vi "Piezo Message Loop.vi"(8 "error in (no error)":errorcluster, 10 "Data Notifiers":T2, 11 "Message Queues":T3) -> (0 "error out":errorcluster)   [LabVIEW 2013, in "Piezo.lvlib"]
uses:
  Piezo.lvlib
  support/Message Queue/All Message Queues.ctl
  support/Message Queue/Message Cluster.ctl
  support/Data Notifiers/All Data Notifiers.ctl
  Acquisition/APD Notifier Cluster.ctl
  Piezo display.ctl
  XY/XY Display.ctl
  Capacitive/Capacitive Signal Cluster.ctl
  Feedback/Error Signal.ctl
  piezo new/Hardware Configuration Piezo NEW.ctl
  Untitled Project 3 Andrea/piezo new/Hardware Configuration Piezo out.ctl
  Piezo State.ctl
  support/Message Queue/Enqueue Message (Single).vi
  <vilib>/Utility/error.llb/Error Cluster From Error Code.vi
  <vilib>/ErrorRing/Error Ring.xnode
  support/Message Queue/Message Queue.lvlib
  Acquisition/Acquisition.lvlib
  XY/XY.lvlib
  support/Data Notifiers/Data Notifiers.lvlib
  Capacitive/Capacitive.lvlib
  Feedback/Feedback.lvlib
panel:
  out "Numeric":i32
  in  "Cluster":T1
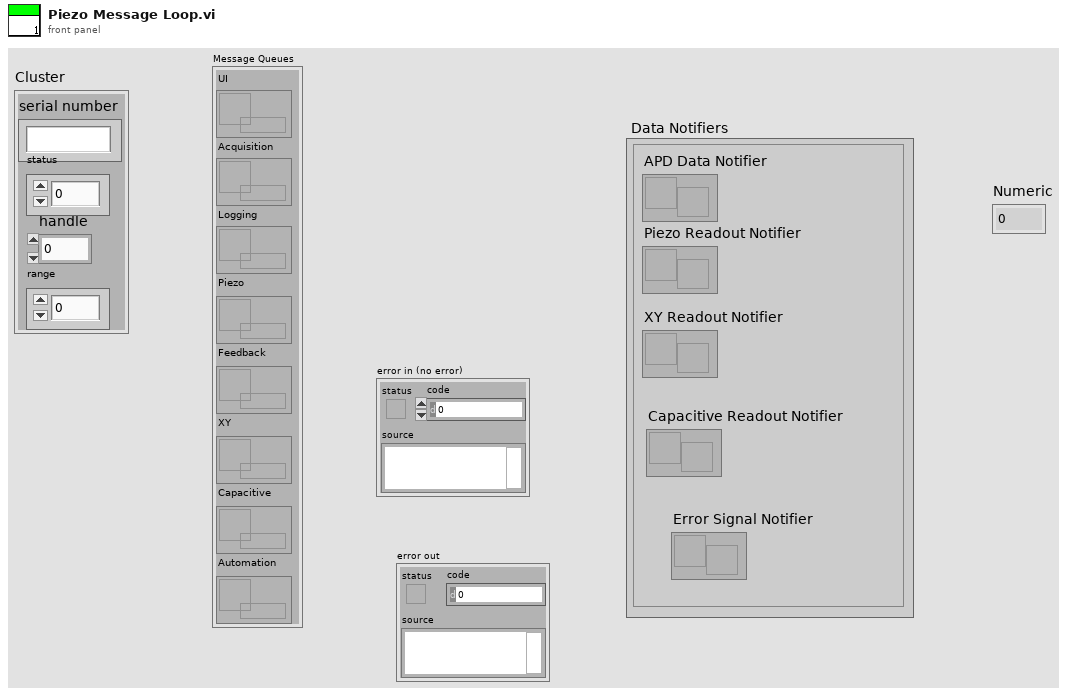
[diagram p1: front panel]
types:
  T1 = typedef "Hardware Configuration Piezo NEW.ctl" = cluster{"serial number":string, "handle":i32, "status":i32, "range":i32}
  T2 = typedef "Data Notifiers.lvlib/All Data Notifiers.ctl" = cluster{"APD Data Notifier":refnum<notifier>, "Piezo Readout Notifier":refnum<notifier>, "XY Readout Notifier":refnum<notifier>, "Capacitive Readout Notifier":refnum<notifier>, "Error Signal Notifier":refnum<notifier>}
  T3 = typedef "Message Queue.lvlib/All Message Queues.ctl" = cluster{"UI":refnum<queue>, "Acquisition":refnum<queue>, "Logging":refnum<queue>, "Piezo":refnum<queue>, "Feedback":refnum<queue>, "XY":refnum<queue>, "Capacitive":refnum<queue>, "Automation":refnum<queue>}
  T4 = typedef "Hardware Configuration Piezo out.ctl" = cluster{"physical channels":tag, "MAX   VOLTAGE":dbl, "MIN   VOLTAGE":dbl}
  T5 = typedef "Piezo.lvlib/Piezo State.ctl" = enum16{"Idle", "Acquiring"}
  T6 = typedef "Acquisition.lvlib/APD Notifier Cluster.ctl" = cluster{"data":dbl[][], "t0":i32}
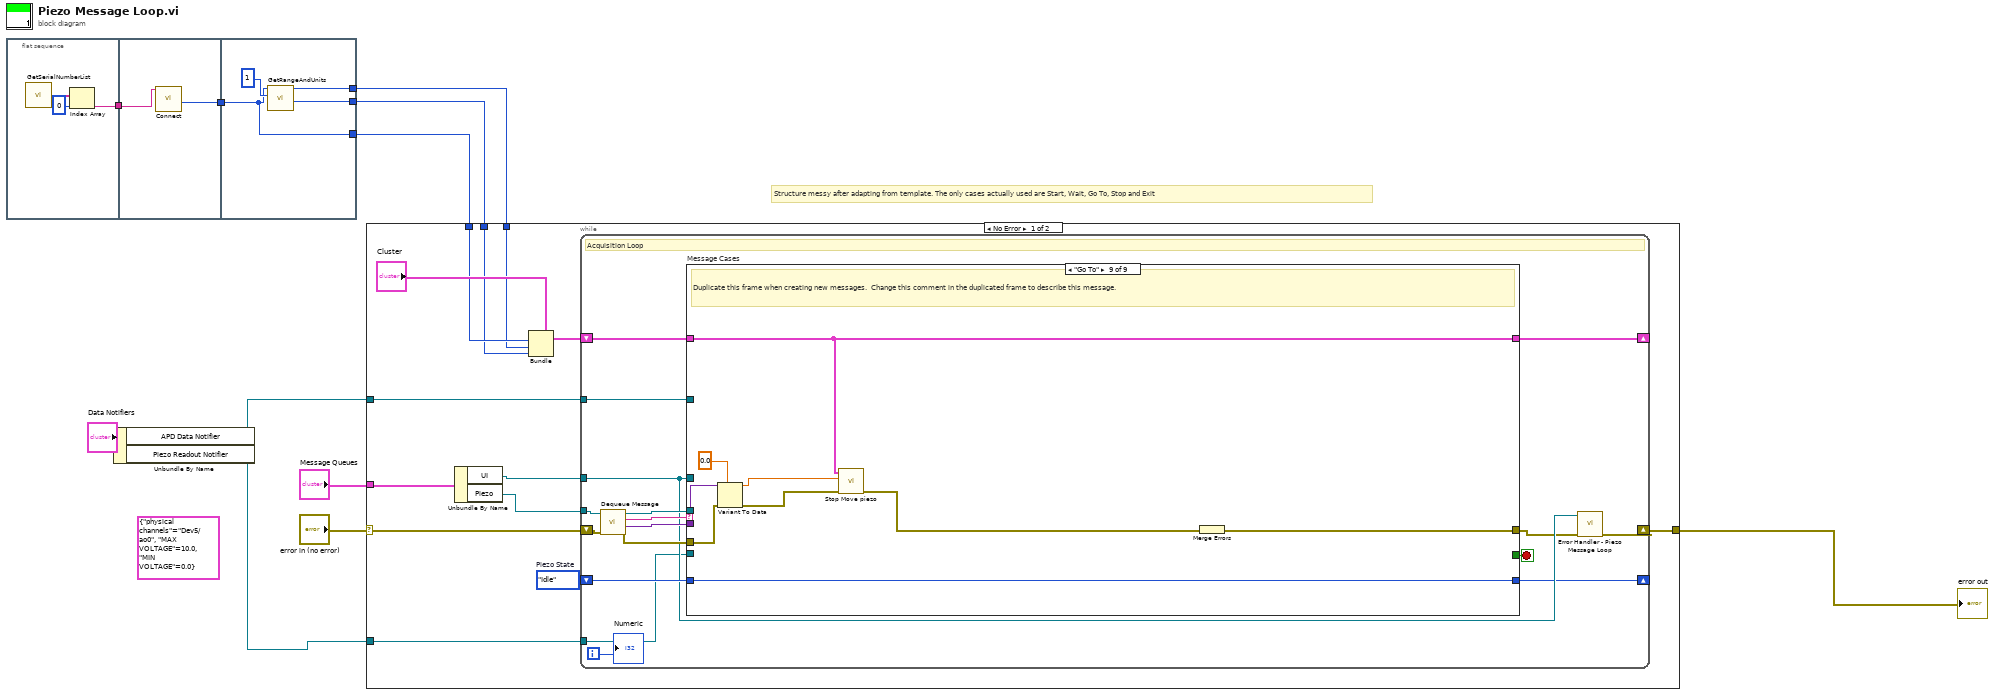
[diagram p0: block diagram]
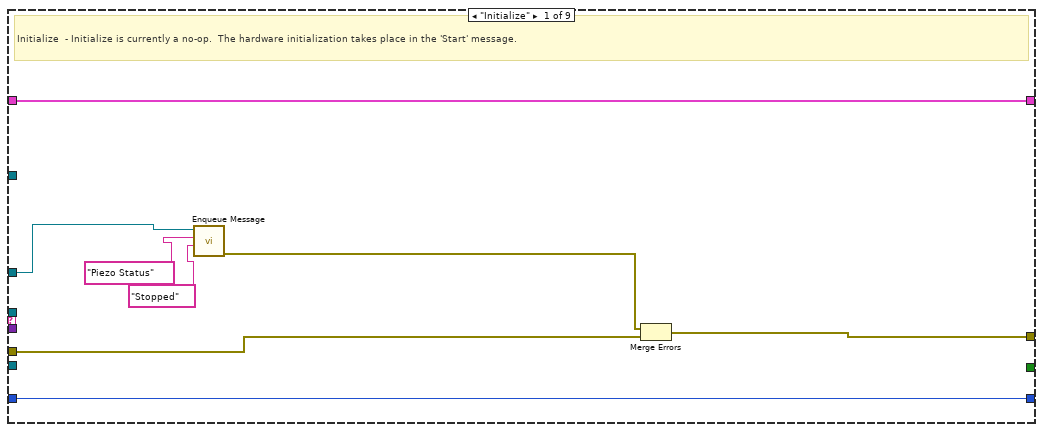
[diagram p2: hidden frame]
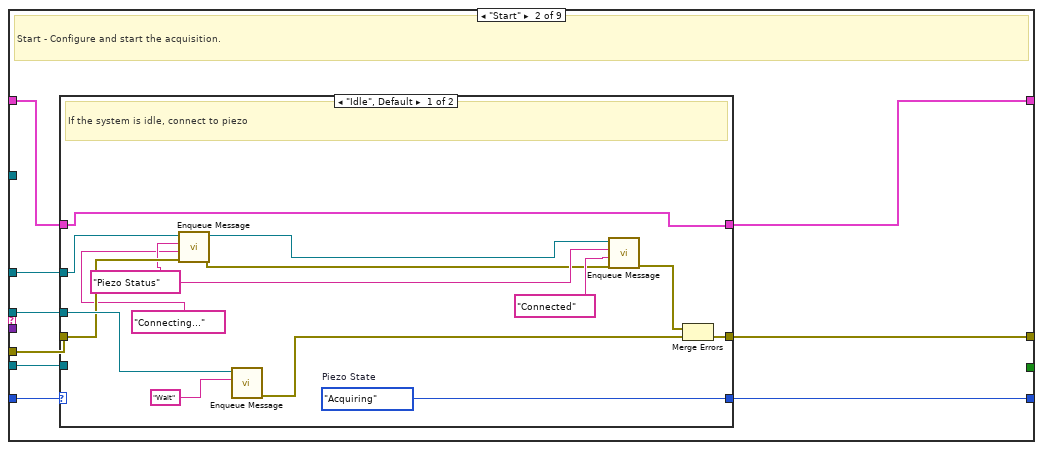
[diagram p3: hidden frame]
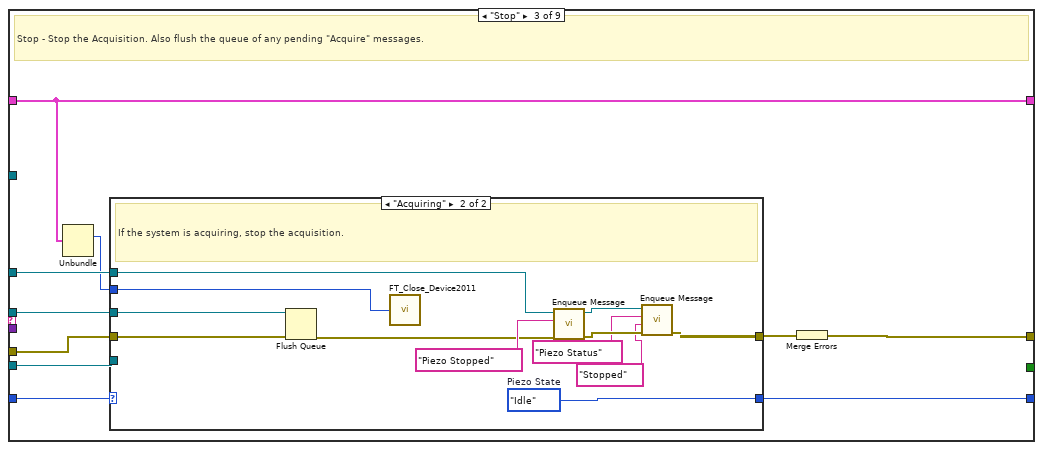
[diagram p5: hidden frame]
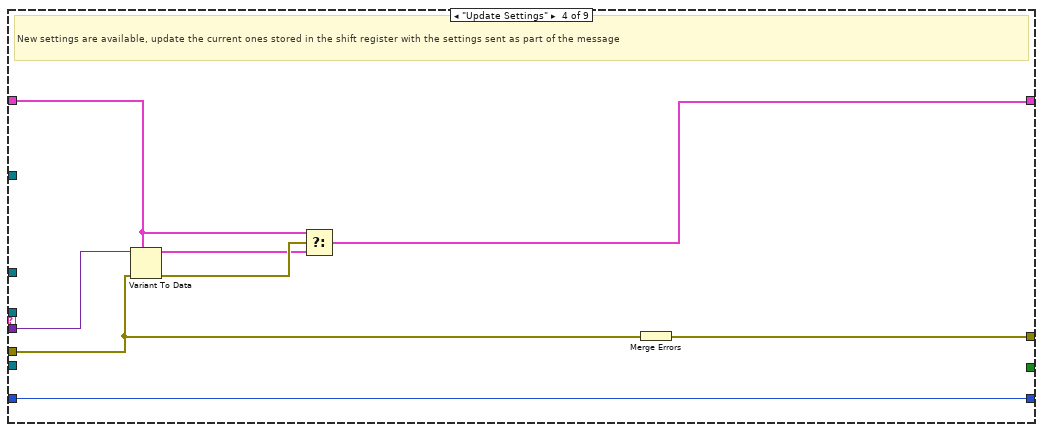
[diagram p7: hidden frame]
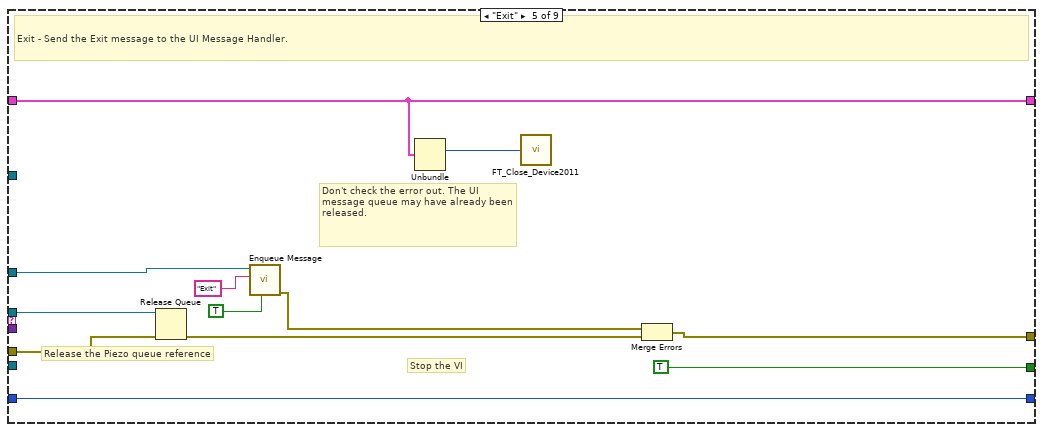
[diagram p8: hidden frame]
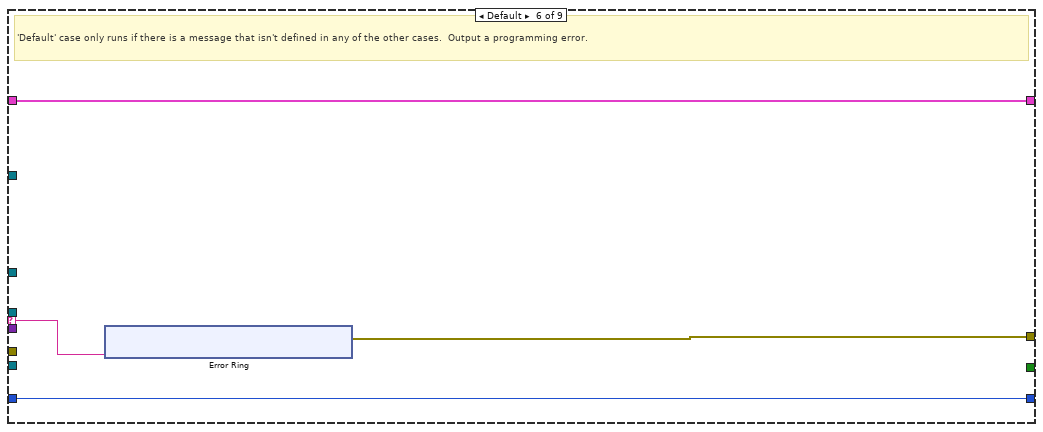
[diagram p9: hidden frame]
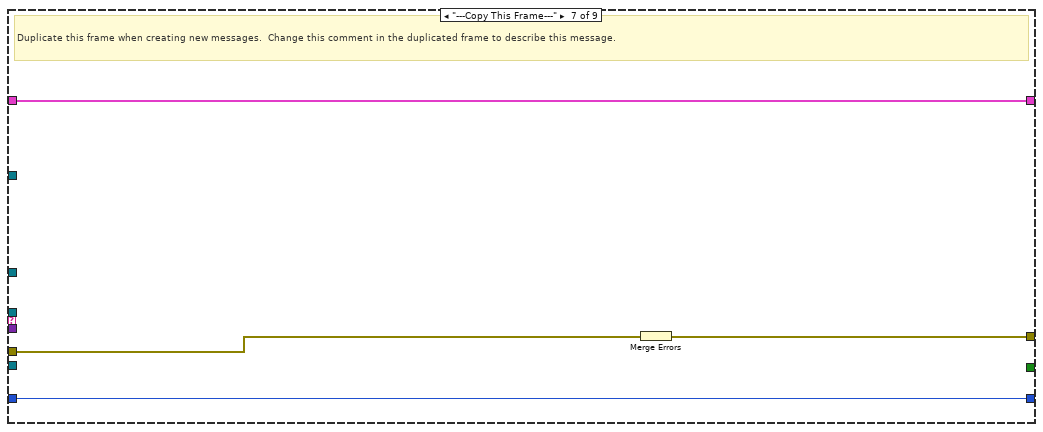
[diagram p10: hidden frame]
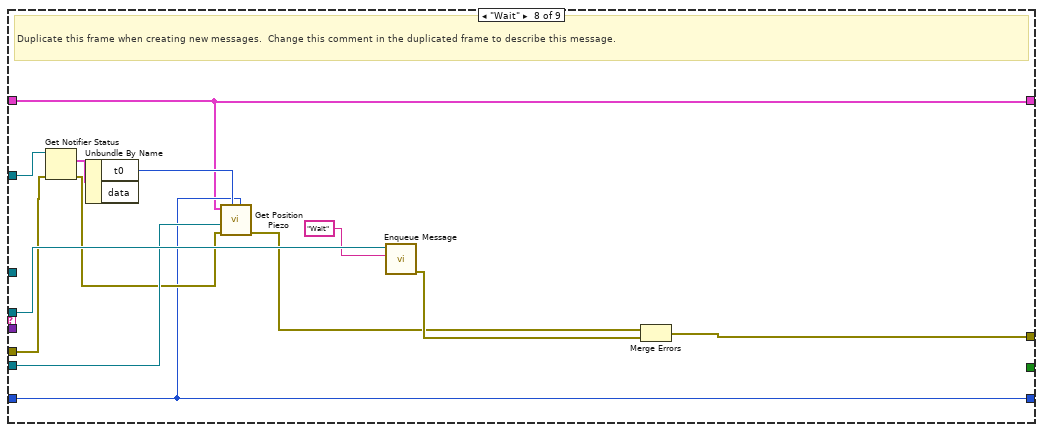
[diagram p11: hidden frame]
diagram:
  (unwired) T4 {"physical channels"="Dev5/ao0", "MAX   VOLTAGE"=10.0, "MIN   VOLTAGE"=0.0} ("Cluster")
  # "Structure messy after adapting from template. The only cases actually used are Start, Wait, Go To, Stop and Exit"
  n1 = flat-sequence {
    tunnel: [w12] -> w5
    tunnel: w5 -> [w16]
    tunnel: [w15] -> w4
    tunnel: w4 -> [w18]
    tunnel: [w19] -> w2
    tunnel: [w18] -> w3
    tunnel: [w17] -> w1
    frame #0 {
      n2 = call "GetSerialNumberList.vi"() -> ("C400 Serial Number Array"=w13:string[])  [unwired: 11 in]
      n3 = Index Array(array=w13, index=0) -> (element=w12:string)
    }
    frame #1 {
      n4 = call "Connect.vi"("Device Serial Number"=w16) -> ("Handle"=w15:u32)  [unwired: 9 in, 1 out]
    }
    frame #2 {
      n5 = call "GetRangeAndUnits.vi"("Handle"=w18, "Controller Channel"=1) -> ("FT_Status"=w17:u32, "Range"=w19:i32)  [unwired: 6 in, 1 out]
    }
  }
  n6 = Unbundle By Name("Data Notifiers") -> ("APD Data Notifier"=w7:refnum<notifier>, "Piezo Readout Notifier"=w6:refnum<notifier>)
  n7 = case shown="No Error" "error in (no error)" {
    selector: "error in (no error)" -> [w28 w166]
    tunnel: "Message Queues" -> [w33 _]
    tunnel: [w31 w166] -> w10
    tunnel: w6 -> [w27 _]
    tunnel: w7 -> [w26 _]
    tunnel: w3 -> [w23 _]
    tunnel: w2 -> [w22 _]
    tunnel: w1 -> [w21 _]
    frame No Error {
      w29 = Piezo_State."Idle"  # Piezo State
      n8 = Unbundle By Name(w33) -> ("UI"=w30:refnum<queue>, "Piezo"=w32:refnum<queue>)
      n9 = Bundle(cluster="Cluster", "handle"=w23, "status"=w21, "range"=w22) -> (w25:T1)  [unwired: 1 in]
      n10 = while {
        tunnel: w32 -> [w43]
        shift-right: [w38] -> _
        shift-left: w25 -> [w50]
        shift-right: [w40] -> w31
        shift-left: w28 -> [w48]
        tunnel: w30 -> [w41]
        shift-right: [w39] -> _
        shift-left: w29 -> [w42]
        tunnel: w27 -> [w36]
        tunnel: w26 -> [w35]
        i -> [w34]
        stop <- w49 stop-if-true
        # "Acquisition Loop"
        n11 = call "Dequeue Message.vi"("error in (no error)"=w48, "Message Queue"=w43) -> ("error out"=w47:errorcluster, "Message Data"=w45:variant, "Message"=w46:string, "dup Message Queue"=w44:refnum<queue>)  [unwired: 6 in]
        n12 = case "Message Cases" shown="\"Go To\"" w46 {
          selector: w46 -> [_ _ _ _ _ w132 _ _ _]
          tunnel: w44 -> [_ w64 w92 _ w124 _ _ w155 _]
          tunnel: w47 -> [w57 w65 w93 w111 w126 _ w143 w152 w161]
          tunnel: [w58 w67 w94 w116 w127 w131 w142 w156 w165] -> w37
          tunnel: w50 -> [w55 w66 w86 w112 w117 w129 w140 w144 w157]
          tunnel: [_ _ _ _ TRUE _ _ _ _] -> w49
          tunnel: w45 -> [_ _ _ w115 _ _ _ _ w163]
          tunnel: w41 -> [w53 w60 w91 _ w120 _ _ _ _]
          tunnel: w42 -> [w56 w63 w90 w110 w123 w130 w141 w146 w164]
          tunnel: [w56 w62 w89 w110 w123 w130 w141 w146 w164] -> w39
          tunnel: [w55 w61 w86 w109 w117 w129 w140 w144 w157] -> w38
          tunnel: w36 -> [_ w59 w87 _ _ _ _ w149 _]
          tunnel: w35 -> [_ _ _ _ _ _ _ w151 _]
          frame "Initialize" {
            # "Initialize  - Initialize is currently a no-op.  The hardware initialization takes place in the 'Start' message."
            n13 = call-poly "Enqueue Message.vi"("Message Data"="Stopped" ("Message"), "Message"="Piezo Status", "Message Queue"=w53) -> ("error out"=w52:errorcluster)  [unwired: 7 in, 1 out]
            n14 = Merge Errors(w52, w57) -> (w58:errorcluster)
          }
          frame "Start" {
            # "Start - Configure and start the acquisition."
            n15 = case shown="\"Idle\", Default" w63 {
              selector: w63 -> [_ w82]
              tunnel: [w81 w84] -> w67
              tunnel: w66 -> [w68 w83]
              tunnel: w65 -> [w73 w84]
              tunnel: w64 -> [w78 _]
              tunnel: [w68 w83] -> w61
              tunnel: [w80 w82] -> w62
              tunnel: w60 -> [w74 _]
              tunnel: w59 -> [_ _]
              frame "Idle", Default {
                w71 = "Piezo Status" ("Message")
                w80 = Piezo_State."Acquiring"  # Piezo State
                # "If the system is idle, connect to piezo"
                n16 = call-poly "Enqueue Message.vi"("error in (no error)"=w73, "Message Data"="Connecting..." ("Message"), "Message"=w71, "Message Queue"=w74) -> ("error out"=w69:errorcluster, "dup Message Queue"=w72:refnum<queue>)  [unwired: 6 in]
                n17 = call-poly "Enqueue Message.vi"("Message"="Wait", "Message Queue"=w78) -> ("error out"=w77:errorcluster)  [unwired: 8 in, 1 out]
                n18 = call-poly "Enqueue Message.vi"("error in (no error)"=w69, "Message Data"="Connected" ("Message"), "Message"=w71, "Message Queue"=w72) -> ("error out"=w76:errorcluster)  [unwired: 6 in, 1 out]
                n19 = Merge Errors(w76, w77) -> (w81:errorcluster)
              }
              frame "Acquiring" {
                # "The system is already acquiring. Ignore the \"Start\" message."
              }
            }
          }
          frame "Stop" {
            # "Stop - Stop the Acquisition. Also flush the queue of any pending \"Acquire\" messages."
            n20 = Unbundle(w86) -> ("handle"=w85:i32)  [unwired: 3 out]
            n21 = case shown="\"Acquiring\"" w90 {
              selector: w90 -> [w96 _]
              tunnel: w93 -> [w95 w99]
              tunnel: w92 -> [_ w108]
              tunnel: w91 -> [_ w107]
              tunnel: [w96 w105] -> w89
              tunnel: [w95 w102] -> w88
              tunnel: w87 -> [_ _]
              tunnel: w85 -> [_ w97]
              frame "Idle", Default {
                # "The system is already idle. Ignore the \"Stop\" message."
              }
              frame "Acquiring" {
                w105 = Piezo_State."Idle"  # Piezo State
                # "If the system is acquiring, stop the acquisition."
                n22 = Flush Queue(queue=w108, error in (no error)=w99) -> (error out=w98:errorcluster)  [unwired: 2 out]
                n23 = call "FT_Close_Device2011.vi"("Handle"=w97) -> ()  [unwired: 1 out]
                n24 = call-poly "Enqueue Message.vi"("error in (no error)"=w98, "Message"="Piezo Stopped", "Message Queue"=w107) -> ("error out"=w103:errorcluster, "dup Message Queue"=w104:refnum<queue>)  [unwired: 7 in]
                n25 = call-poly "Enqueue Message.vi"("error in (no error)"=w103, "Message Data"="Stopped" ("Message"), "Message"="Piezo Status", "Message Queue"=w104) -> ("error out"=w102:errorcluster)  [unwired: 6 in, 1 out]
              }
            }
            n26 = Merge Errors(w88) -> (w94:errorcluster)
          }
          frame "Update Settings" {
            # "New settings are available, update the current ones stored in the shift register with the settings sent as part of the message"
            n27 = Variant To Data(error in=w111, type=w112, Variant=w115) -> (data=w113:T1, error out=w114:errorcluster)
            n28 = Select(t=w112, s=w114, f=w113) -> (s? t:f=w109:T1)
            n29 = Merge Errors(w111) -> (w116:errorcluster)
          }
          frame "Exit" {
            # "Don't check the error out. The UI message queue may have already been released."
            # "Release the Piezo queue reference"
            # "Stop the VI"
            # "Exit - Send the Exit message to the UI Message Handler."
            n30 = Release Queue(queue=w124, error in (no error)=w126) -> (error out=w125:errorcluster)  [unwired: 1 in, 2 out]
            n31 = call-poly "Enqueue Message.vi"("Priority Message? (F)"=TRUE, "Message"="Exit", "Message Queue"=w120) -> ("error out"=w119:errorcluster)  [unwired: 7 in, 1 out]
            n32 = Unbundle(w117) -> ("handle"=w118:i32)  [unwired: 3 out]
            n33 = call "FT_Close_Device2011.vi"("Handle"=w118) -> ()  [unwired: 1 out]
            n34 = Merge Errors(w119, w125) -> (w127:errorcluster)
          }
          frame Default {
            # "'Default' case only runs if there is a message that isn't defined in any of the other cases.  Output a programming error."
            n35 = xnode "Error Ring"("parameter 0"=w132) -> ("error out"=w131:errorcluster)
          }
          frame "---Copy This Frame---" {
            # "Duplicate this frame when creating new messages.  Change this comment in the duplicated frame to describe this message."
            n36 = Merge Errors(w143) -> (w142:errorcluster)
          }
          frame "Wait" {
            # "Duplicate this frame when creating new messages.  Change this comment in the duplicated frame to describe this message."
            n37 = Get Notifier Status(notifier=w151, error in (no error)=w152) -> (current notification=w150:T6, error out=w148:errorcluster)  [unwired: 3 out]
            n38 = Unbundle By Name(w150) -> ("t0"=w147:i32)  [unwired: 1 out]
            n39 = call "Get Position Piezo.vi"("Piezo State"=w146, "Counter Time"=w147, "error in (no error)"=w148, "notifier out"=w149, "Cluster 3"=w144) -> ("error out"=w145:errorcluster)  [unwired: 6 in]
            n40 = call-poly "Enqueue Message.vi"("Message"="Wait", "Message Queue"=w155) -> ("error out"=w153:errorcluster)  [unwired: 8 in, 1 out]
            n41 = Merge Errors(w145, w153) -> (w156:errorcluster)
          }
          frame "Go To" {
            # "Duplicate this frame when creating new messages.  Change this comment in the duplicated frame to describe this message."
            n42 = Variant To Data(error in=w161, type=sgl 0.0, Variant=w163) -> (data=w160:sgl, error out=w159:errorcluster)
            n43 = call "Stop Move piezo.vi"("error in (no error)"=w159, "MOVE TO [MICRON]"=w160, "Cluster 2"=w157) -> ("error out"=w158:errorcluster)  [unwired: 8 in]
            n44 = Merge Errors(w158) -> (w165:errorcluster)
          }
        }
        n45 = call "Error Handler - Piezo Message Loop.vi"("error in (no error)"=w37, "Message Queue"=w41) -> ("dup error in"=w40:errorcluster)  [unwired: 8 in, 1 out]
        "Numeric" <- w34
      }
    }
    frame Error {
    }
  }
  "error out" <- w10
